vi "PH_PPMA_PowerUnit.src Wait for Shot Cmd.vi"(0 "i ref in":refnum<vi>, 5 "error in (no error)":errorcluster) -> (14 "i ref out":refnum<vi>, 19 "error out":errorcluster)   [LabVIEW 2014, in "PH_PPMA_PowerUnit.lvlib"]
doc: "This is the action VI of the Shot event case. It checks the state of the SM and related Devices. If\n\nState SM = \"Wait for Shot Cmd\",\nWaiting Time over? = true,\nState Rel Rods = off (DumpRods down), \nState PSU = off, \nState PSU = off,and\nIgnitron.State Device = on,\nthen a request state change is send to the SM to get \"Open DumpRods\"."
uses:
  PH_PPMA_PowerUnit.lvlib
  PH_Basics/PH_StatusHandler/PH_StatusHandler.Status.ctl
  PH_Basics/PH_PowerUnit_BaseClass/PH_PowerUnit_BaseClass.SM States.ctl
  PH_Basics/PH_PowerUnit_BaseClass/PH_PowerUnit_BaseClass.lvlib
  PH_Basics/PH_StatusHandler/PH_StatusHandler.lvlib
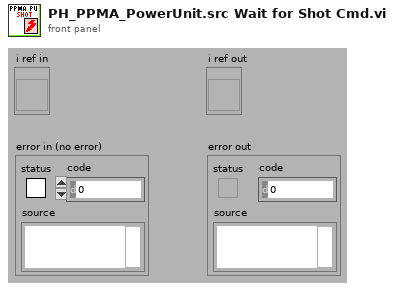
[diagram p1: front panel]
types:
  T1 = typedef "PH_PowerUnit_BaseClass.lvlib/PH_PowerUnit_BaseClass.SM States.ctl" = enum16{".", "Stand by", "Switch PU on", "Configure", "Set Default Voltage", "Set STANDBY", "Set READY", "Wait for Shot Cmd", "Open Dump Rods", "Open Ross Relais", "Close Ross Relais", "Switch PSU on", "Switch PSU off", "Charge", "Switch GD Channel on", "Close Dump Rods", "Rods-TO", "RR-TO", "PSU-TO", "Trigger-TO"}
  T2 = typedef "PH_StatusHandler.lvlib/PH_StatusHandler.Status.ctl" = i16
  T3 = typedef "PH_PPMA_PowerUnit.lvlib/PH_PPMA_PowerUnit.i attribute.ctl" = cluster{"GUI Refs":cluster{"Rods":refnum<vi>, "Ignitron":refnum<vi>, "Rossrelais":refnum<vi>, "Set Voltage":refnum<vi>, "PSU":refnum<vi>, "EOC":refnum<vi>, "Trigger":refnum<vi>}, "Rods":T4, "PSU":T5, "Ross Relais":T6, "Ignitron":T7, "Trigger":cluster{"State Device":T2, "linked?":bool}, "Timing Settings":cluster{"Prdc Fast?":bool, "Default Value Periodic Interval":i32, "Mercury on since":dbl, "Warm up Time Mercury [s]":dbl}, "Set Voltage [V]":dbl}
  T4 = typedef "PH_PPMA_PowerUnit.lvlib/PH_PPMA_PowerUnit.Rods Attributes.ctl" = cluster{"Instancename":string, "Device Status":T2, "linked?":bool}
  T5 = typedef "PH_PP_Common.lvlib/PH_PP_Common.PSU Attributes.ctl" = cluster{"lower limit [V]":dbl, "upper limit [V]":dbl, "Voltage set":bool, "State Device":T2, "linked?":bool}
  T6 = typedef "PH_PP_Common.lvlib/PH_PP_Common.Ross Relais Attributes.ctl" = cluster{"State Device":T2, "linked?":bool}
  T7 = typedef "PH_PP_Common.lvlib/PH_PP_Common.Ignitron Attributes.ctl" = cluster{"State Device":T2, "linked?":bool}
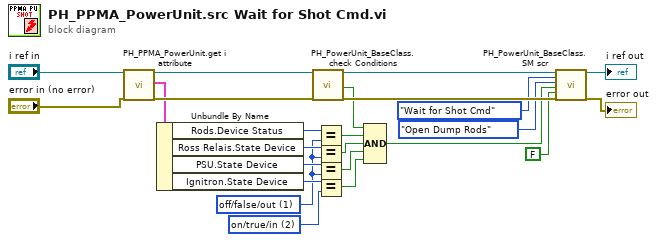
[diagram p0: block diagram]
diagram:
  w11 = T2 2 items=["no info", "off/false/out", "on/true/in", "Failure", "Alarm", "Status 1", "Status 2", "Status 3"] ("Ignitron.State Device")
  w12 = T2 1 items=["no info", "off/false/out", "on/true/in", "Failure", "Alarm", "Status 1", "Status 2", "Status 3"] ("PSU.State PSU")
  n1 = call "PH_PPMA_PowerUnit.get i attribute.vi"("i ref in"="i ref in", "error in (no error)"="error in (no error)") -> ("i ref out"=w9:refnum<vi>, "i attribute"=w21:T3, "error out"=w24:errorcluster)  [unwired: 15 in]
  n2 = Unbundle By Name(w21) -> ("Rods.Device Status"=w20:T2, "Ross Relais.State Device"=w18:T2, "PSU.State Device"=w17:T2, "Ignitron.State Device"=w14:T2)
  n3 = call "PH_PowerUnit_BaseClass.check Conditions.vi"("VI in"=w9, "error in (no error)"=w24) -> ("VI out"=w8:refnum<vi>, "Ready for shot"=w7:bool, "error out"=w10:errorcluster)  [unwired: 14 in, 1 out]
  n4 = Equal?(x=w20, y=w12) -> (x = y?=w19:bool)
  n5 = Equal?(x=w18, y=w12) -> (x = y?=w16:bool)
  n6 = Equal?(x=w17, y=w12) -> (x = y?=w15:bool)
  n7 = Equal?(x=w14, y=w11) -> (x = y?=w13:bool)
  n8 = Compound Arithmetic op=AND(w7, w19, w16, w15, w13) -> (w6:bool)
  n9 = call "PH_PowerUnit_BaseClass.SM scr.vi"("VI in"=w8, "Current SM State (condition)"=PH_PowerUnit_BaseClass.SM_States."Wait for Shot Cmd", "Wanted SM State"=PH_PowerUnit_BaseClass.SM_States."Open Dump Rods", "Further change condition"=w6, "PU in use is condition? (true)"=FALSE, "error in (no error)"=w10) -> ("VI out"=→"i ref out":refnum<vi>, "error out"=→"error out":errorcluster)  [unwired: 12 in]
